vi "S2C_FORNAX_Poly_UserSettingsCommand.vi"(8 "Error In":errorcluster, 10 "UserSettingsCommand":T3={"Partition"="Default", "Message"="UserSettingsCommand", "M_UserSetting"=0, "M_Command"=0, "M_IntValue"=0, "M_StringValue"=""} {"M_Command" items=["USER_SETTINGS_COMMAND_NONE", "USER_SETTINGS_COMMAND_WRITE", "USER_SETTINGS_COMMAND_READ", "USER_SETTINGS_COMMAND_RESTORE_TO_DEFAULT"]; "M_UserSetting" items=["USER_SETTINGS_INVALID", "USER_SETTINGS_LANGUAGE", "USER_SETTINGS_VOLUME", "USER_SETTINGS_ALIAS", "USER_SETTINGS_NETWORK_CONFIG", "USER_SETTINGS_AUTO_NETWORK_ON", "USER_SETTINGS_KEYBOARD_LANGUAGE", "NUM_USER_SETTINGS"]}, 11 "Settings":T4={"Driver"="Fornax", "Command"="UserSettingsCommand", "Return"="ErrorStatus", "Parameters"="", "Timeout"=10.0}) -> (0 "Error Out":errorcluster, 3 "Response":string)   [LabVIEW 2015]
uses:
  Typedefs/UserSettings.ctl
  Typedefs/UserSettingsCommand.ctl
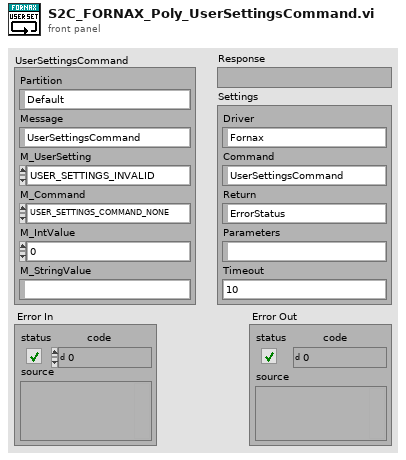
[diagram p1: front panel]
types:
  T1 = typedef "UserSettings.ctl" = i16
  T2 = typedef "UserSettingsCommand.ctl" = i16
  T3 = cluster{"Partition":string, "Message":string, "M_UserSetting":T1, "M_Command":T2, "M_IntValue":i32, "M_StringValue":string}
  T4 = cluster{"Driver":string, "Command":string, "Return":string, "Parameters":string, "Timeout":dbl}
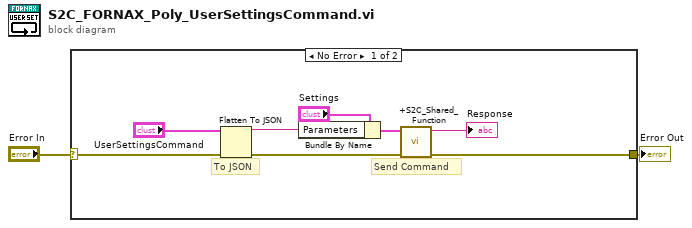
[diagram p0: block diagram]
diagram:
  n1 = case shown="No Error" "Error In" {
    selector: "Error In" -> [w6 w11]
    tunnel: [w5 w11] -> w1
    frame No Error {
      # "To JSON"
      # "Send Command"
      n2 = Flatten To JSON(anything="UserSettingsCommand", error in (no error)=w6) -> (JSON string=w7:string, 11:w9:errorcluster)  [unwired: 1 in]
      n3 = Bundle By Name(cluster="Settings", "Parameters"=w7) -> (w10:T4)
      n4 = call "+S2C_Shared_Function.vi"("Error In"=w9, "Settings"=w10) -> ("Error Out"=w5:errorcluster, "Response"=→"Response":string)  [unwired: 8 in]
    }
    frame Error {
    }
  }
  "Error Out" <- w1
